vi "BRig_dataTrial_tSelection.vi"() -> (2 "output_tSelection":i32)   [LabVIEW 2014]
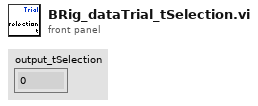
[diagram p1: front panel]
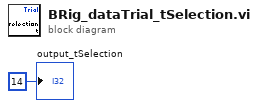
[diagram p0: block diagram]
diagram:
  "output_tSelection" <- 14 ("output_iBlock")
